vi "GT Ln XYZACUVW.vi"(0 "cardNum":i16, 1 "synVel":dbl, 2 "velEnd":dbl, 5 "crd":i16, 7 "pPos":i32, 9 "posMask":i16, 11 "error in (no error)":errorcluster caption="错误输入（无错误）", 12 "synAcc":dbl, 13 "fifo":i16) -> (4 "function return":i16, 8 "pPos out":i32, 15 "error out":errorcluster caption="错误输出")   [LabVIEW 2014, in "gts.lvlib"]
doc: "GT_API GT_LnXYZACUVW(short cardNum,short crd,long *pPos,short posMask,double synVel,double synAcc,double velEnd=0,short fifo=0);"
uses:
  gts.lvlib
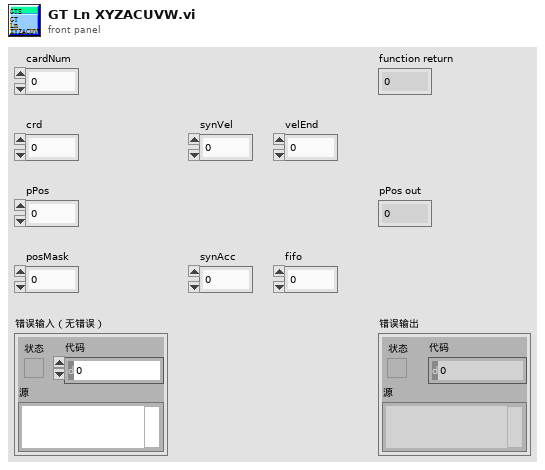
[diagram p1: front panel]
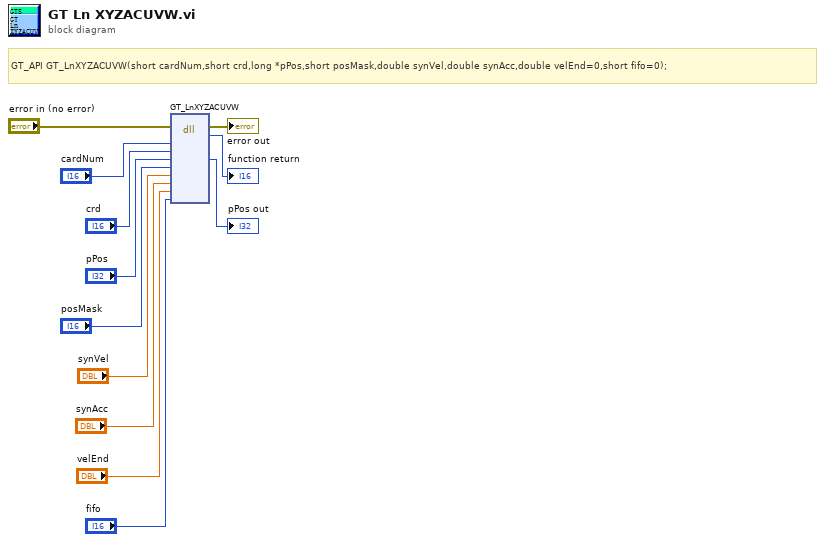
[diagram p0: block diagram]
diagram:
  # "GT_API GT_LnXYZACUVW(short cardNum,short crd,long *pPos,short posMask,double synVel,double synAcc,double velEnd=0,short fifo=0);"
  n1 = dll-call lib="PTH2habs D固高科技资料GTS控制卡GTS卡18年上半年资料dllVC32bit\nmulti_cardgts.*" fn="GT_LnXYZACUVW"(error in="error in (no error)", "cardNum"="cardNum", "crd"="crd", "pPos"="pPos", "posMask"="posMask", "synVel"="synVel", "synAcc"="synAcc", "velEnd"="velEnd", "fifo"="fifo") -> (error out=→"error out":errorcluster, →"function return":i16, "pPos"=→"pPos out":i32)  [unwired: 9 in, 1 out]
